vi "Start Edge Drag.vi"(0 "FSM in":refnum<class "FSM.Graph.lvclass">, 7 "Dragged nodes":string[](array[string]), 9 "Grid size":dbl, 11 "error in (no error)":errorcluster) -> (4 "FSM out":refnum<class "FSM.Graph.lvclass">, 15 "error out":errorcluster)   [LabVIEW 2015, in "FSM.Graph.lvclass"]
uses:
  FSM.Graph.lvclass
  FSM.Graph.lvclass/FSM.Graph.ctl
  FSM.Edge/FSM.Edge.lvclass
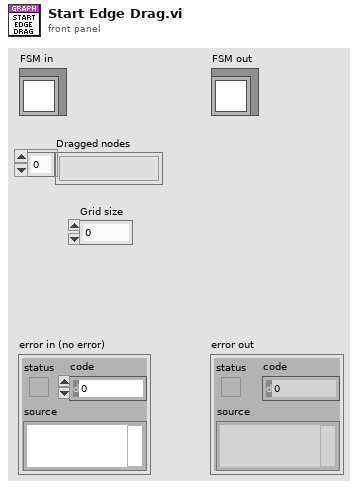
[diagram p1: front panel]
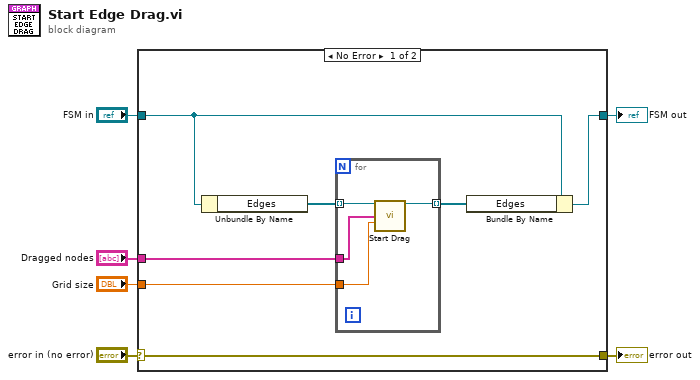
[diagram p0: block diagram]
diagram:
  n1 = case shown="No Error" "error in (no error)" {
    selector: "error in (no error)" -> [w13 w19]
    tunnel: [w13 w19] -> w5
    tunnel: [w10 w18] -> w3
    tunnel: "FSM in" -> [w12 w18]
    tunnel: "Dragged nodes" -> [w8 _]
    tunnel: "Grid size" -> [w7 _]
    frame No Error {
      n2 = Unbundle By Name(w12) -> ("Edges"=w11:refnum<class "FSM.Edge.lvclass">[])
      n3 = for {
        tunnel: w8 -> [w16]
        tunnel: w11 -> [w17] mode=indexing
        tunnel: [w15] -> w9 mode=indexing
        tunnel: w7 -> [w14]
        n4 = call "Start Drag.vi"("FSM.Edge in"=w17, "dragged nodes"=w16, "Grid size"=w14) -> ("FSM.Edge out"=w15:refnum<class "FSM.Edge.lvclass">)  [unwired: 12 in]
      }
      n5 = Bundle By Name(cluster=w12, "Edges"=w9) -> (w10:refnum<class "FSM.Graph.lvclass">)
    }
    frame Error {
    }
  }
  "error out" <- w5
  "FSM out" <- w3
